vi "SetDefaults.vi"(8 "error in (no error)":errorcluster, 11 "LoggingWrapper in":refnum<class "LoggingWrapper.lvclass">) -> (0 "error out":errorcluster, 3 "LoggingWrapper out":refnum<class "LoggingWrapper.lvclass">)   [LabVIEW 2022 SP3, in "Logger.lvlib" / "LoggingWrapper.lvclass"]
uses:
  LoggingWrapper.lvclass
  LoggingWrapper.lvclass/LoggingWrapper.ctl
  PythonWrapper/Source/PythonWrapper/PythonWrapper.lvclass
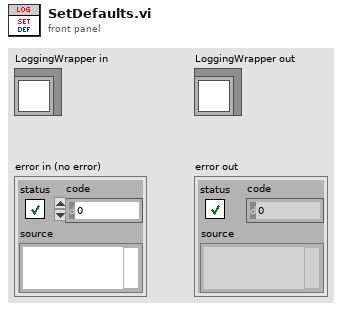
[diagram p1: front panel]
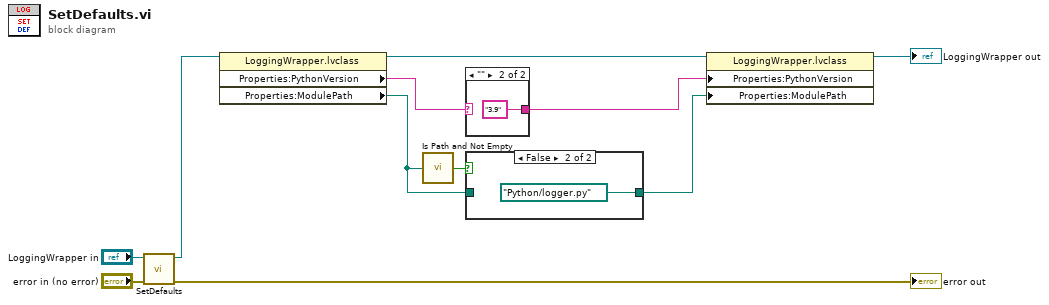
[diagram p0: block diagram]
diagram:
  n1 = call-parent "SetDefaults.vi"("error in (no error)"="error in (no error)", "PythonWrapper in"="LoggingWrapper in") -> ("error out"=→"error out":errorcluster, "PythonWrapper out"=w1:refnum<class "LoggingWrapper.lvclass">)  [unwired: 8 in]
  n2 = property class="LoggingWrapper.lvclass"(reference=w1) -> (reference out=w8:refnum<class "LoggingWrapper.lvclass">, "Properties:PythonVersion"=w7:string, "Properties:ModulePath"=w4:path)  [unwired: 1 in, 1 out]
  n3 = call <vilib>:"Is Path and Not Empty.vi"("path"=w4) -> ("Is Path and Not Empty?"=w5:bool)  [unwired: 4 in]
  n4 = case shown="\"\"" w7 {
    selector: w7 -> [w12 _]
    tunnel: [w12 "3.9"] -> w6
    frame Default {
    }
    frame "" {
    }
  }
  n5 = case shown="False" w5 {
    tunnel: [w14 path "Python/logger.py" ("Properties:ModulePath")] -> w3
    tunnel: w4 -> [w14 _]
    frame True {
    }
    frame False {
    }
  }
  n6 = property class="LoggingWrapper.lvclass"(reference=w8, "Properties:PythonVersion"=w6, "Properties:ModulePath"=w3) -> (reference out=→"LoggingWrapper out":refnum<class "LoggingWrapper.lvclass">)  [unwired: 1 in, 1 out]
